vi "Search New Tweets - Continuous.vi"() -> ()   [LabVIEW 2011]
doc: "An example that continuously searches for a Query on Twitter"
uses:
  Controls/Tweet.ctl
  SubVIs/Twitter Open - Desktop.vi
  i3-twitter.lvlib
panel:
  in  "Query":string
  in  "Consumer Secret":string
  in  "Consumer Key":string
  in  "Num of Tweets to Read":i32
  out "Num of Tweets Read":i32
  out "Time Stamp of Newest Tweet":timestamp
  in  "stop":bool
  out "Tweets Read":T1[](array[typedef])
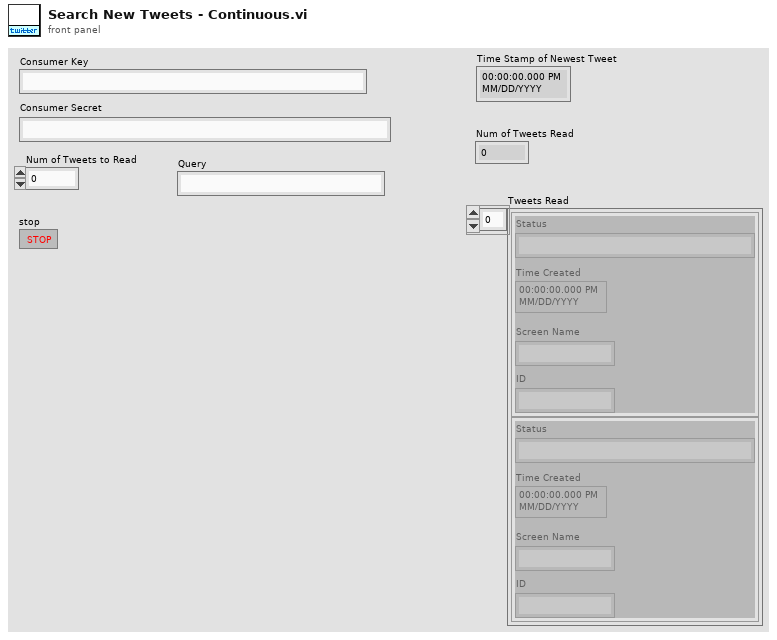
[diagram p1: front panel]
types:
  T1 = typedef "i3-twitter.lvlib/Tweet.ctl" = cluster{"Status":string, "Time Created":timestamp, "Screen Name":string, "ID":string}
  T2 = typedef "i3-oauth.lvlib/Credentials.ctl" = cluster{"Token":string, "Secret":string}
  T3 = typedef "i3-twitter.lvlib/Twitter Handle.ctl" = cluster{"OAuth Credentials":T4, "since ID":string, "max ID":string, "Screen Name":string}
  T4 = typedef "i3-oauth.lvlib/OAuth Handle.ctl" = cluster{"Signature Method":T5, "Version":string, "Client":T2, "Access":T2}
  T5 = typedef "i3-oauth.lvlib/Signature Method.ctl" = enum16{"HMAC-MD5", "HMAC-SHA1", "HMAC-SHA224", "HMAC-SHA256", "HMAC-SHA384", "HMAC-SHA512"}
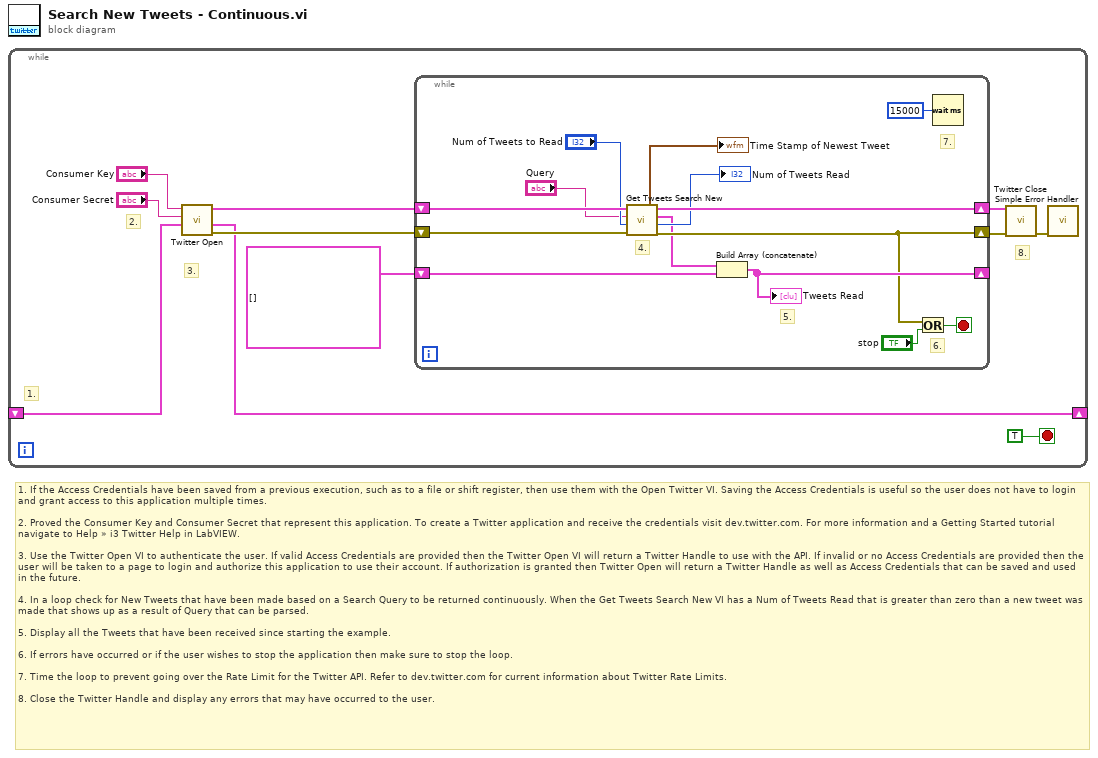
[diagram p0: block diagram]
diagram:
  # "1. If the Access Credentials have been saved from a previous execution, such as to a file or shift register, then use them with the Open Twitter VI. Saving the Access Credentials is useful so the user does not have to login and grant access to this application multiple times.\n\n2. Proved the Consumer Key and Consumer Secret that represent this application. To create a Twitter application and receive the credentials visit dev.twitter.com. For more information and a Getting Started tutorial navigate to Help » i3 Twitter Help in LabVIEW.\n\n3. Use the Twitter Open VI to authenticate the user. If valid Access Credentials are provided then the Twitter Open VI will return a Twitter Handle to use with the API. If invalid or no Access Credentials are provided then the user will be taken to a page to login and authorize this application to use their account. If authorization is granted then Twitter Open will return a Twitter Handle as well as Access Credentials that can be saved and used in the future.\n\n4. In a loop check for New Tweets that have been made based on a Search Query to be returned continuously. When the Get Tweets Search New VI has a Num of Tweets Read that is greater than zero than a new tweet was made that shows up as a result of Query that can be parsed.\n\n5. Display all the Tweets that have been received since starting the example.\n\n6. If errors have occurred or if the user wishes to stop the application then make sure to stop the loop.\n\n7. Time the loop to prevent going over the Rate Limit for the Twitter API. Refer to dev.twitter.com for current information about Twitter Rate Limits.\n\n8. Close the Twitter Handle and display any errors that may have occurred to the user."
  n1 = while {
    shift-right: [w2] -> _
    shift-left: _ -> [w1]
    stop <- TRUE stop-if-true
    # "8."
    # "3."
    # "2."
    # "1."
    n2 = call-poly "Twitter Open.vi"("Access Credentials (in)"=w1, "Consumer Secret"="Consumer Secret", "Consumer Key"="Consumer Key") -> ("error out"=w5:errorcluster, "Access Credentials (out)"=w2:T2, "Twitter Handle Out"=w9:T3)  [unwired: 6 in]
    n3 = while {
      shift-right: [w23] -> w7
      shift-left: w9 -> [w25]
      shift-right: [w21] -> _
      shift-left: T1[] [] ("Tweets Array") -> [w14]
      shift-right: [w18] -> w8
      shift-left: w5 -> [w24]
      stop <- w17 stop-if-true
      # "7."
      # "6."
      # "5."
      # "4."
      n4 = call "Get Tweets Search New.vi"("error in"=w24, "Tweets to Read (10)"="Num of Tweets to Read", "Query"="Query", "Twitter Handle In"=w25) -> ("error out"=w18:errorcluster, "Actual Num of Tweets Read"=→"Num of Tweets Read":i32, "New Tweets Read"=w15:T1[], "Twitter Handle Out"=w23:T3, "Time Stamp of Newest Tweet"=→"Time Stamp of Newest Tweet":timestamp)  [unwired: 3 in]
      n5 = Build Array (concatenate)(w15, w14) -> (w21:T1[])
      "Tweets Read" <- w21
      n6 = Or(x=w18, y="stop") -> (x .or. y?=w17:bool)
      n7 = Wait (ms)(milliseconds to wait=u32 15000) -> ()  [unwired: 1 out]
    }
    n8 = call "Twitter Close.vi"("error in"=w8, "Twitter Handle In"=w7) -> ("error in"=w3:errorcluster)  [unwired: 9 in]
    n9 = call <vilib>:"Simple Error Handler.vi"("error in (no error)"=w3) -> ()  [unwired: 4 in, 5 out]
  }
